vi "test_RS-xxx Write.vi"(8 "error in (no error)":errorcluster, 11 "TestCase in":refnum<class "Serial Protocols Tests.lvclass">) -> (0 "error out":errorcluster, 3 "TestCase out":refnum<class "Serial Protocols Tests.lvclass">)   [LabVIEW 2019, in "Serial Protocols Tests.lvclass"]
uses:
  Serial Protocols Tests.lvclass
  Listener/Listener.lvclass
  Listener/ListenerClassControls/Operation.ctl
  RS-xxx/RS-xxx.lvclass
  D:/GitRepository/niveristand-instrument-addon-classes/Source/Protocols/Protocol Parent/Protocol Parent.lvclass
  <vilib>/Platform/TimedLoop/XDataNode/timing_clust.ctl
  <vilib>/Platform/TimedLoop/XDataNode/nitl_modes.ctl
  <vilib>/Platform/TimedLoop/XDataNode/wakeup.ctl
  RS-xxx/RS-xxx.lvclass/RS-xxx.ctl
  <vilib>/platform/TimedLoop/XDataNode/XDataNode.xnode
  <vilib>/addons/_JKI Toolkits/VI Tester/TestCase.llb/TestCase.lvclass
  <vilib>/Platform/TimedLoop/XDataNode/XDNodeRunTimeDep.lvlib
  C:/Program Files (x86)/National Instruments/LabVIEW 2019/vi.lib/addons/_JKI Toolkits/VI Tester/TestCase.llb/TestCase.lvclass
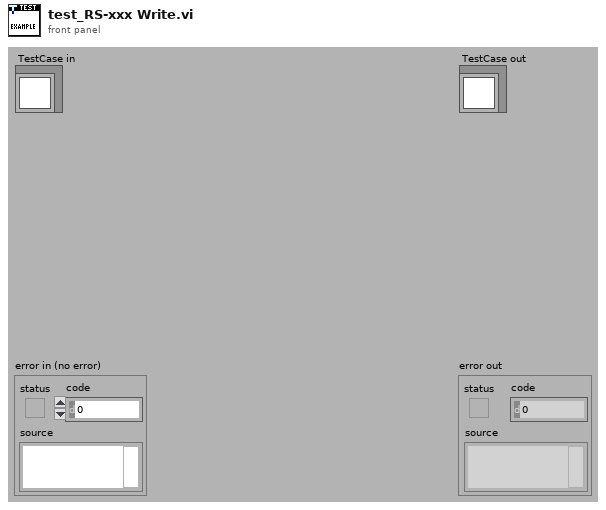
[diagram p1: front panel]
types:
  T1 = typedef "Listener.lvclass/Operation.ctl" = enum16{"Read", "Write"}
  T2 = typedef "XDNodeRunTimeDep.lvlib/timing_clust.ctl" = cluster{"Expected End [f-1]":u64, "Actual End [f-1]":u64, "Finished Late? [f-1]":bool, "Expected End [i-1]":u64, "Actual End [i-1]":u64, "Finished Late? [i-1]":bool, "Expected Start [i]":u64, "Actual Start [i]":u64, "Expected Start [f]":u64, "Actual Start [f]":u64, "Source Name":string, "Structure Name":string, "Period":i64, "Deadline":i64, "Offset":i64, "Start":i64, "Priority":i32, "Timeout":i32, "Mode":T3, "Wakeup Reason":T4, "Error":errorcluster, "Source Type":string, "Secondary Source Type":string, "Global End Time":u64, "Global Start Time":u64, "Frame Duration":u64, "Iteration Duration":u64, "Assigned CPU":i32, "I/O Scan Engine Mode":u32}
  T3 = typedef "XDNodeRunTimeDep.lvlib/nitl_modes.ctl" = enum32{"No Change", "Process missed periods, maintain original phase", "Discard missed periods, maintain original phase", "Process missed periods, ignore original phase", "Discard missed periods, ignore original phase"}
  T4 = typedef "XDNodeRunTimeDep.lvlib/wakeup.ctl" = enum32{"Normal", "Aborted", "Asynchronous wakeup", "Timing source error", "Timed loop error", "Timeout"}
  T5 = typedef "Listener.lvclass/RS-xxx Data Structure.ctl" = cluster{"Protocol Port Ref":refnum<visa-resource-name>, "Listener Port Ref":refnum<visa-resource-name>, "Virtual COM Port Settings 1":cluster{"Port":string, "Baud Rate":u32, "Data Bits":u16, "Parity":enum16{"None", "Odd", "Even", "Mark", "Space"}, "Stop Bits":u16, "Flow Control":u16, "XON":enum16{"NUL", "SOH", "STX", "ETX", "EOT", "ENQ", "ACK", "BEL", "BS", "HT", "LF", "VT", "FF", "CR", "SO", "SI", "DLE", "DC1", "DC2", "DC3", "DC4", "NAK", "SYN", "ETB", "CAN", "EM", "SUB", "ESC", "FS", "GS", "RS", "US", "SP", "!", "\"", "#", "$", "%", "&", "'", "(", ")", "*", "+", ",", "- (-)", ".", "/", "0", "1", "2", "3", "4", "5", "6", "7", "8", "9", ":", ";", "<", "=", ">", "?", "@", "A", "B", "C", "D", "E", "F", "G", "H", "I", "J", "K", "L", "M", "N", "O", "P", "Q", "R", "S", "T", "U", "V", "W", "X", "Y", "Z", "[", "\\", "]", "^", "_", "`", "a", "b", "c", "d", "e", "f", "g", "h", "i", "j", "k", "l", "m", "n", "o", "p", "q", "r", "s", "t", "u", "v", "w", "x", "y", "z", "{", "|", "}", "~"}, "XOFF":enum16{"NUL", "SOH", "STX", "ETX", "EOT", "ENQ", "ACK", "BEL", "BS", "HT", "LF", "VT", "FF", "CR", "SO", "SI", "DLE", "DC1", "DC2", "DC3", "DC4", "NAK", "SYN", "ETB", "CAN", "EM", "SUB", "ESC", "FS", "GS", "RS", "US", "SP", "!", "\"", "#", "$", "%", "&", "'", "(", ")", "*", "+", ",", "- (-)", ".", "/", "0", "1", "2", "3", "4", "5", "6", "7", "8", "9", ":", ";", "<", "=", ">", "?", "@", "A", "B", "C", "D", "E", "F", "G", "H", "I", "J", "K", "L", "M", "N", "O", "P", "Q", "R", "S", "T", "U", "V", "W", "X", "Y", "Z", "[", "\\", "]", "^", "_", "`", "a", "b", "c", "d", "e", "f", "g", "h", "i", "j", "k", "l", "m", "n", "o", "p", "q", "r", "s", "t", "u", "v", "w", "x", "y", "z", "{", "|", "}", "~"}, "End Read on Termination Character":bool, "End Write on Termination Character":bool, "Termination Character":u8}, "Virtual COM Port Settings 2":cluster{"Port":string, "Baud Rate":u32, "Data Bits":u16, "Parity":enum16{"None", "Odd", "Even", "Mark", "Space"}, "Stop Bits":u16, "Flow Control":u16, "XON":enum16{"NUL", "SOH", "STX", "ETX", "EOT", "ENQ", "ACK", "BEL", "BS", "HT", "LF", "VT", "FF", "CR", "SO", "SI", "DLE", "DC1", "DC2", "DC3", "DC4", "NAK", "SYN", "ETB", "CAN", "EM", "SUB", "ESC", "FS", "GS", "RS", "US", "SP", "!", "\"", "#", "$", "%", "&", "'", "(", ")", "*", "+", ",", "- (-)", ".", "/", "0", "1", "2", "3", "4", "5", "6", "7", "8", "9", ":", ";", "<", "=", ">", "?", "@", "A", "B", "C", "D", "E", "F", "G", "H", "I", "J", "K", "L", "M", "N", "O", "P", "Q", "R", "S", "T", "U", "V", "W", "X", "Y", "Z", "[", "\\", "]", "^", "_", "`", "a", "b", "c", "d", "e", "f", "g", "h", "i", "j", "k", "l", "m", "n", "o", "p", "q", "r", "s", "t", "u", "v", "w", "x", "y", "z", "{", "|", "}", "~"}, "XOFF":enum16{"NUL", "SOH", "STX", "ETX", "EOT", "ENQ", "ACK", "BEL", "BS", "HT", "LF", "VT", "FF", "CR", "SO", "SI", "DLE", "DC1", "DC2", "DC3", "DC4", "NAK", "SYN", "ETB", "CAN", "EM", "SUB", "ESC", "FS", "GS", "RS", "US", "SP", "!", "\"", "#", "$", "%", "&", "'", "(", ")", "*", "+", ",", "- (-)", ".", "/", "0", "1", "2", "3", "4", "5", "6", "7", "8", "9", ":", ";", "<", "=", ">", "?", "@", "A", "B", "C", "D", "E", "F", "G", "H", "I", "J", "K", "L", "M", "N", "O", "P", "Q", "R", "S", "T", "U", "V", "W", "X", "Y", "Z", "[", "\\", "]", "^", "_", "`", "a", "b", "c", "d", "e", "f", "g", "h", "i", "j", "k", "l", "m", "n", "o", "p", "q", "r", "s", "t", "u", "v", "w", "x", "y", "z", "{", "|", "}", "~"}, "End Read on Termination Character":bool, "End Write on Termination Character":bool, "Termination Character":u8}, "Data":string, "Data Length":u32}
  T6 = cluster{"Port":string, "Baud Rate":u32, "Data Bits":u16, "Parity":enum16{"None", "Odd", "Even", "Mark", "Space"}, "Stop Bits":u16, "Flow Control":u16, "XON":enum16{"NUL", "SOH", "STX", "ETX", "EOT", "ENQ", "ACK", "BEL", "BS", "HT", "LF", "VT", "FF", "CR", "SO", "SI", "DLE", "DC1", "DC2", "DC3", "DC4", "NAK", "SYN", "ETB", "CAN", "EM", "SUB", "ESC", "FS", "GS", "RS", "US", "SP", "!", "\"", "#", "$", "%", "&", "'", "(", ")", "*", "+", ",", "- (-)", ".", "/", "0", "1", "2", "3", "4", "5", "6", "7", "8", "9", ":", ";", "<", "=", ">", "?", "@", "A", "B", "C", "D", "E", "F", "G", "H", "I", "J", "K", "L", "M", "N", "O", "P", "Q", "R", "S", "T", "U", "V", "W", "X", "Y", "Z", "[", "\\", "]", "^", "_", "`", "a", "b", "c", "d", "e", "f", "g", "h", "i", "j", "k", "l", "m", "n", "o", "p", "q", "r", "s", "t", "u", "v", "w", "x", "y", "z", "{", "|", "}", "~"}, "XOFF":enum16{"NUL", "SOH", "STX", "ETX", "EOT", "ENQ", "ACK", "BEL", "BS", "HT", "LF", "VT", "FF", "CR", "SO", "SI", "DLE", "DC1", "DC2", "DC3", "DC4", "NAK", "SYN", "ETB", "CAN", "EM", "SUB", "ESC", "FS", "GS", "RS", "US", "SP", "!", "\"", "#", "$", "%", "&", "'", "(", ")", "*", "+", ",", "- (-)", ".", "/", "0", "1", "2", "3", "4", "5", "6", "7", "8", "9", ":", ";", "<", "=", ">", "?", "@", "A", "B", "C", "D", "E", "F", "G", "H", "I", "J", "K", "L", "M", "N", "O", "P", "Q", "R", "S", "T", "U", "V", "W", "X", "Y", "Z", "[", "\\", "]", "^", "_", "`", "a", "b", "c", "d", "e", "f", "g", "h", "i", "j", "k", "l", "m", "n", "o", "p", "q", "r", "s", "t", "u", "v", "w", "x", "y", "z", "{", "|", "}", "~"}, "End Read on Termination Character":bool, "End Write on Termination Character":bool, "Termination Character":u8}
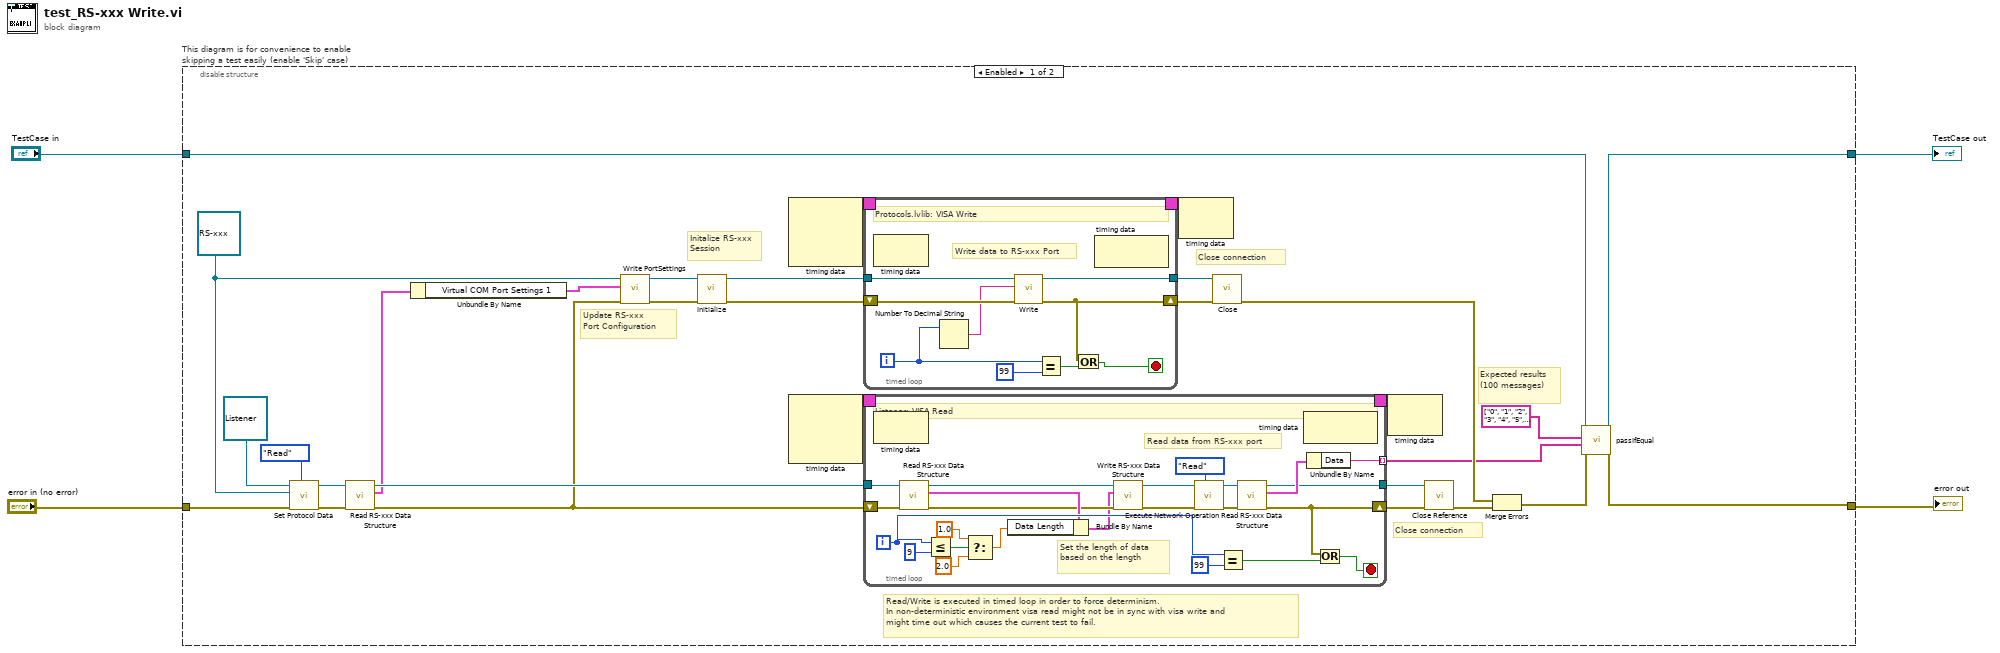
[diagram p0: block diagram]
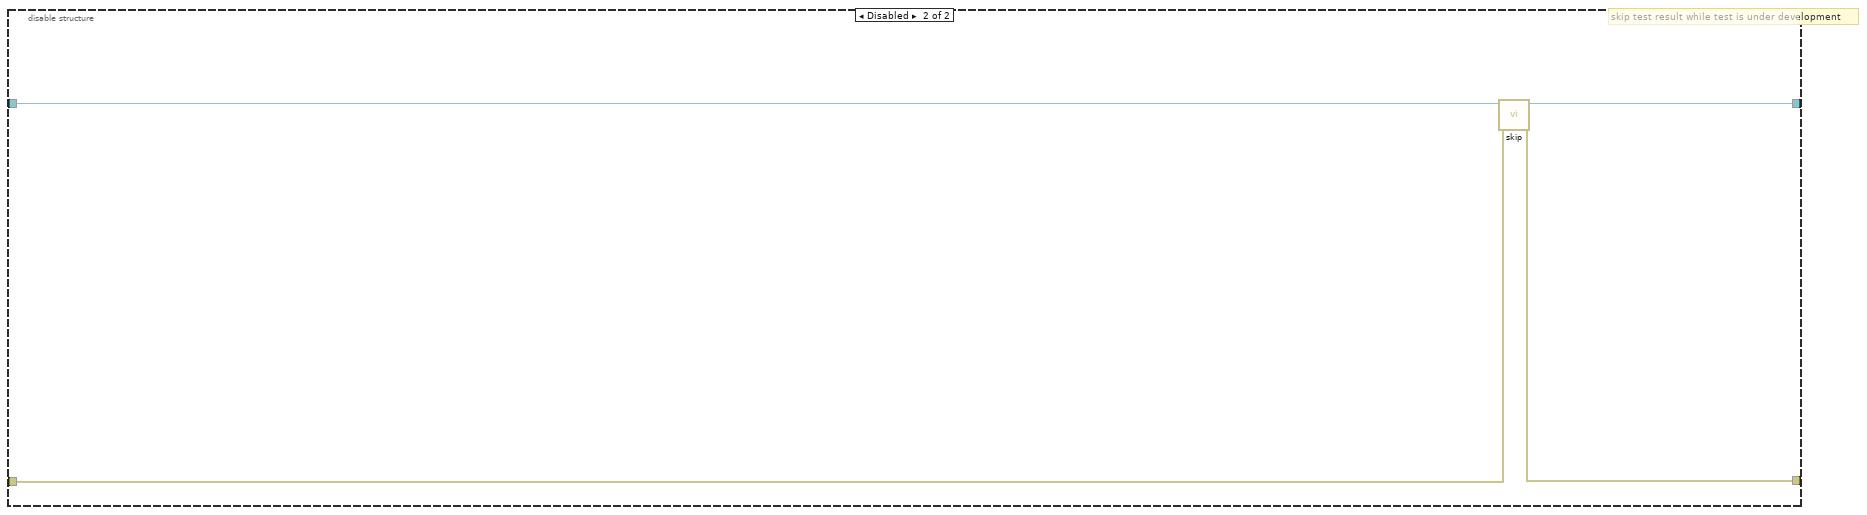
[diagram p2: hidden frame]
diagram:
  n1 = disable-structure "This diagram is for convenience to enable skipping a test easily (enable 'Skip' case)" shown="Enabled" {
    disable-tunnel: "TestCase in" -> [w34 w79]
    disable-tunnel: [w33 w77] -> w1
    disable-tunnel: [w32 w78] -> w3
    disable-tunnel: "error in (no error)" -> [w28 w76]
    frame Enabled {
      w12 = refnum<class "RS-xxx.lvclass"> refnum ("Protocols.lvlib:RS-xxx.lvclass")
      # "Update RS-xxx \nPort Configuration"
      # "Initalize RS-xxx\nSession"
      # "Close connection"
      # "Close connection"
      # "Read/Write is executed in timed loop in order to force determinism.\nIn non-deterministic environment visa read might not be in sync with visa write and\nmight time out which causes the current test to fail."
      # "Expected results\n(100 messages)"
      n2 = call "Set Protocol Data.vi"("Operation"=Operation."Read", "error in (no error)"=w28, "Protocols.lvlib:Protocol Parent.lvclass"=w12, "Listener In.lvclass"=refnum<class "Listener.lvclass"> refnum ("Listener.lvclass")) -> ("error out"=w14:errorcluster, "Listener Out.lvclass"=w15:refnum<class "Listener.lvclass">)  [unwired: 6 in]
      n3 = call-dynamic "Read RS-xxx Data Structure.vi"("error in (no error)"=w14, "Listener in"=w15) -> ("error out"=w7:errorcluster, "RS-xxx Data Structure"=w6:T5, "Listener out"=w8:refnum<class "Listener.lvclass">)  [unwired: 7 in]
      n4 = Unbundle By Name(w6) -> ("Virtual COM Port Settings 1"=w5:T6)
      n5 = call "Write PortSettings.vi"("error in (no error)"=w7, "Cluster"=w5, "RS232 in"=w12) -> ("error out"=w13:errorcluster, "RS232 out"=w11:refnum<class "RS-xxx.lvclass">)  [unwired: 7 in]
      n6 = call-dynamic "Initialize.vi"("error in (no error)"=w13, "RS232 in"=w11) -> ("error out"=w10:errorcluster, "RS232 out"=w9:refnum<class "RS-xxx.lvclass">)  [unwired: 8 in]
      n7 = node-c288() -> (w19:T2)  [unwired: 3 in]
      n8 = node-c288() -> (w17:T2)  [unwired: 3 in]
      n9 = timed-loop {
        shift-right: [w67] -> w23
        shift-left: w10 -> [w66]
        tunnel: [w65] -> w22
        timing: w19 -> [_]
        timing-out: [_] -> w18
        tunnel: w9 -> [w64]
        i -> [w70]
        stop <- w68 stop-if-true
        # "Write data to RS-xxx Port"
        # "Protocols.lvlib: VISA Write"
        n10 = node-c288() -> ()  [unwired: 1 in, 1 out]
        n11 = Number To Decimal String(number=w70) -> (decimal integer string=w63:string)  [unwired: 1 in]
        n12 = call-dynamic "Write.vi"("error in (no error)"=w66, "String"=w63, "RS232 in"=w64) -> ("error out"=w67:errorcluster, "RS232 out"=w65:refnum<class "RS-xxx.lvclass">)  [unwired: 7 in]
        n13 = Equal?(x=w70, y=99) -> (x = y?=w71:bool)
        n14 = Or(x=w67, y=w71) -> (x .or. y?=w68:bool)
        n15 = node-c288() -> ()  [unwired: 1 in, 1 out]
      }
      n16 = timed-loop {
        shift-right: [w46] -> w20
        shift-left: w7 -> [w43]
        tunnel: [w44] -> w21
        tunnel: [w58] -> w25 mode=indexing
        timing: w17 -> [_]
        timing-out: [_] -> w16
        tunnel: w8 -> [w42]
        i -> [w52]
        stop <- w49 stop-if-true
        # "Set the length of data \nbased on the length"
        # "Read data from RS-xxx port"
        # "Listener: VISA Read"
        n17 = node-c288() -> ()  [unwired: 1 in, 1 out]
        n18 = call-dynamic "Read RS-xxx Data Structure.vi"("error in (no error)"=w43, "Listener in"=w42) -> ("error out"=w39:errorcluster, "RS-xxx Data Structure"=w41:T5, "Listener out"=w38:refnum<class "Listener.lvclass">)  [unwired: 7 in]
        n19 = Less Or Equal?(x=w52, y=9) -> (x <= y?=w55:bool)
        n20 = Select(t=1.0, s=w55, f=2.0) -> (s? t:f=w40:dbl)
        n21 = Bundle By Name(cluster=w41, "Data Length"=w40) -> (w37:T5)
        n22 = call-dynamic "Write RS-xxx Data Structure.vi"("error in (no error)"=w39, "RS-xxx Data Structure"=w37, "Listener in"=w38) -> ("error out"=w36:errorcluster, "Listener out"=w35:refnum<class "Listener.lvclass">)  [unwired: 7 in]
        n23 = call "Execute Network Operation.vi"("Operation"=Operation."Read", "error in (no error)"=w36, "Listener In.lvclass"=w35) -> ("error out"=w48:errorcluster, "Listener Out.lvclass"=w47:refnum<class "Listener.lvclass">)  [unwired: 7 in]
        n24 = Equal?(x=w52, y=99) -> (x = y?=w50:bool)
        n25 = call-dynamic "Read RS-xxx Data Structure.vi"("error in (no error)"=w48, "Listener in"=w47) -> ("error out"=w46:errorcluster, "RS-xxx Data Structure"=w45:T5, "Listener out"=w44:refnum<class "Listener.lvclass">)  [unwired: 7 in]
        n26 = node-c288() -> ()  [unwired: 1 in, 1 out]
        n27 = Unbundle By Name(w45) -> ("Data"=w58:string)
        n28 = Or(x=w46, y=w50) -> (x .or. y?=w49:bool)
      }
      n29 = node-c288(w18) -> ()  [unwired: 1 out]
      n30 = call-dynamic "Close.vi"("error in (no error)"=w23, "RS232 in"=w22) -> ("error out"=w27:errorcluster)  [unwired: 8 in, 1 out]
      n31 = node-c288(w16) -> ()  [unwired: 1 out]
      n32 = call "Close Reference.vi"("error in (no error)"=w20, "Listener In.lvclass"=w21) -> ("error out"=w26:errorcluster)  [unwired: 9 in]
      n33 = Merge Errors(w27, w26) -> (w29:errorcluster)
      n34 = call-dynamic "passIfEqual.vi"("error in (no error)"=w29, "y"=w25, "x"=string[] ["0", "1", "2", "3", "4", "5", "6", "7", "8", "9", "10", "11", "12", "13", "14", "15", "16", "17", "18", "19", "20", "21", "22", "23", "24", "25", "26", "27", "28", "29", "30", "31", "32", "33", "34", "35", "36", "37", "38", "39", "40", "41", "42", "43", "44", "45", "46", "47", "48", "49", "50", "51", "52", "53", "54", "55", "56", "57", "58", "59", "60", "61", "62", "63", "64", "65", "66", "67", "68", "69", "70", "71", "72", "73", "74", "75", "76", "77", "78", "79", "80", "81", "82", "83", "84", "85", "86", "87", "88", "89", "90", "91", "92", "93", "94", "95", "96", "97", "98", "99"] ("Array"), "TestCase in"=w34) -> ("error out"=w32:errorcluster, "TestCase out"=w33:refnum<class "Serial Protocols Tests.lvclass">)  [unwired: 6 in]
    }
    frame Disabled {
      # "skip test result while test is under development"
      n35 = call <vilib>:"skip.vi"("error in (no error)"=w76, "TestCase in"=w79) -> ("error out"=w78:errorcluster, "TestCase out"=w77:refnum<class "Serial Protocols Tests.lvclass">)  [unwired: 8 in]
    }
  }
  "error out" <- w3
  "TestCase out" <- w1
